vi "MH_LibVersion_global.vi"() -> ()   [LabVIEW 2010]
panel:
  in  "Library Version":string="3.1"
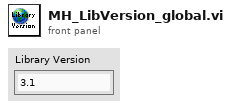
[diagram p1: front panel]
diagram:
